vi "Handle Zoom on GPU.vi"(7 "FFT Size / 2 in":u64, 8 "error in (no error)":errorcluster, 9 "element":T1 {"Zoom Parameters"."fwidth:" format="%#_6p"; "Zoom Parameters"."f0:" format="%#_6p"}, 10 "df":dbl, 11 "Unzoomed Data In":refnum<class "2D Array f32.lvclass">) -> (0 "error out":errorcluster, 1 "Zoomed Size":u64, 2 "f0:":dbl, 3 "Zoomed Data Out":refnum<class "2D Array f32.lvclass">)   [LabVIEW 2020, in "GPU FFT Calculator.lvlib" / "GPU FFT Calculator.lvclass"]
uses:
  GPU FFT Calculator.lvclass
  GPU Calculation Message.ctl
  <vilib>/Natan Biesmans/G2CPU GPU and CPU HPC Toolkit/G2CPU Libraries/Async IO/DMA Manager/DMA Manager.lvclass
  <vilib>/Natan Biesmans/G2CPU GPU and CPU HPC Toolkit/G2CPU Libraries/Arrays/1DArray/s16/1D Array s16.lvclass
  <vilib>/Natan Biesmans/G2CPU GPU and CPU HPC Toolkit/G2CPU Libraries/Arrays/1DArray/f32/1D Array f32.lvclass
  chart zoom.ctl
  GPU Metrics.ctl
  <vilib>/Natan Biesmans/G2CPU GPU and CPU HPC Toolkit/G2CPU Libraries/Arrays/2DArray/f32/2D Array f32.lvclass
  C:/Program Files/National Instruments/LabVIEW 2026/vi.lib/Natan Biesmans/G2CPU GPU and CPU HPC Toolkit/G2CPU Libraries/Arrays/Array/Array Prototype.lvclass
  <vilib>/Natan Biesmans/G2CPU GPU and CPU HPC Toolkit/G2CPU Libraries/Arrays/Array/Array Prototype.lvclass/Array Prototype.ctl
  8252e44e-a382-477c-9ca7-689a626c88eb.vi
  e1576fc2-ceb6-43a4-8527-5ba273ea8d14.vi
  ddde6bd1-7626-4236-9c85-82b4f95f97b4.vi
  8252e44e-a382-477c-9ca7-689a626c88eb.vi/ab6cfe59-c8ad-4da3-839b-8d02ec9e015f.vi
  <vilib>/Natan Biesmans/G2CPU GPU and CPU HPC Toolkit/G2CPU Libraries/Arrays/Array/G2CPU Get Array Pointer.vi
  e1576fc2-ceb6-43a4-8527-5ba273ea8d14.vi/5793b77b-c002-4ebf-9075-685617c95341.vi
  e1576fc2-ceb6-43a4-8527-5ba273ea8d14.vi/2ed3ef86-c00d-4d71-b84c-20267a6dfcf9.vi
  ddde6bd1-7626-4236-9c85-82b4f95f97b4.vi/2e03f477-51b7-4ba0-bb4f-4f838f6557e6.vi
  ddde6bd1-7626-4236-9c85-82b4f95f97b4.vi/125d45d4-836b-469d-8a4a-6adb452f866d.vi
  ddde6bd1-7626-4236-9c85-82b4f95f97b4.vi/8038e9ed-2e71-4568-91ba-0d873494c5ed.vi
  8252e44e-a382-477c-9ca7-689a626c88eb.vi/ab6cfe59-c8ad-4da3-839b-8d02ec9e015f.vi/313ec8c5-c203-475c-9de0-0583f6fb8b4d.vi
  e1576fc2-ceb6-43a4-8527-5ba273ea8d14.vi/5793b77b-c002-4ebf-9075-685617c95341.vi/3e802c67-fb96-46a3-ae13-4994a8508b4f.vi
  e1576fc2-ceb6-43a4-8527-5ba273ea8d14.vi/5793b77b-c002-4ebf-9075-685617c95341.vi/5a50fc67-79e7-4972-80c2-92243cd53dd4.vi
  e1576fc2-ceb6-43a4-8527-5ba273ea8d14.vi/5793b77b-c002-4ebf-9075-685617c95341.vi/1c928fc9-710a-40e7-8c4f-08a1069452ae.vi
  e1576fc2-ceb6-43a4-8527-5ba273ea8d14.vi/2ed3ef86-c00d-4d71-b84c-20267a6dfcf9.vi/730f6c57-5c0b-4ee9-b61e-75067b25222b.vi
  e1576fc2-ceb6-43a4-8527-5ba273ea8d14.vi/2ed3ef86-c00d-4d71-b84c-20267a6dfcf9.vi/096b8799-7810-404e-baca-ba9279cec4bd.vi
  e1576fc2-ceb6-43a4-8527-5ba273ea8d14.vi/2ed3ef86-c00d-4d71-b84c-20267a6dfcf9.vi/0f1a5a47-bcc5-4796-ac31-8dfcfbc0d7d1.vi
  e1576fc2-ceb6-43a4-8527-5ba273ea8d14.vi/2ed3ef86-c00d-4d71-b84c-20267a6dfcf9.vi/89f12e17-3330-4b72-ad8f-8dd636660732.vi
  ddde6bd1-7626-4236-9c85-82b4f95f97b4.vi/2e03f477-51b7-4ba0-bb4f-4f838f6557e6.vi/d8e2d9cc-c923-495e-b121-b6b84788c73f.vi
  ddde6bd1-7626-4236-9c85-82b4f95f97b4.vi/2e03f477-51b7-4ba0-bb4f-4f838f6557e6.vi/345e91f0-9a5e-4de4-af9c-133346717e4a.vi
  <vilib>/Natan Biesmans/G2CPU GPU and CPU HPC Toolkit/ArrayFire Driver/VIs/Run as Multi Device.vi
  e1576fc2-ceb6-43a4-8527-5ba273ea8d14.vi/5793b77b-c002-4ebf-9075-685617c95341.vi/3e802c67-fb96-46a3-ae13-4994a8508b4f.vi/1b7cf390-2ae0-48f3-9bce-03c57eed6ee8.vi
  <vilib>/Natan Biesmans/G2CPU GPU and CPU HPC Toolkit/G2CPU Libraries/Arrays/1DArray/u32/1D Array u32.lvclass
  <vilib>/Natan Biesmans/G2CPU GPU and CPU HPC Toolkit/G2CPU Libraries/Arrays/1DArray/s32/1D Array s32.lvclass
  <vilib>/Natan Biesmans/G2CPU GPU and CPU HPC Toolkit/ArrayFire Driver/VIs/range.vi
  <vilib>/Natan Biesmans/G2CPU GPU and CPU HPC Toolkit/G2CPU Libraries/Arrays/Array/G2CPU Set Array Pointer.vi
  <vilib>/Natan Biesmans/G2CPU GPU and CPU HPC Toolkit/ArrayFire Driver/subvi/Error Converter (ErrCode or Status).vi
  <vilib>/Natan Biesmans/G2CPU GPU and CPU HPC Toolkit/G2CPU Libraries/Arrays/SubVI/is 1D.vi
  <vilib>/Natan Biesmans/G2CPU GPU and CPU HPC Toolkit/ArrayFire Driver/VIs/add.vi
  <vilib>/Natan Biesmans/G2CPU GPU and CPU HPC Toolkit/ArrayFire Driver/VIs/cast.vi
  <vilib>/Natan Biesmans/G2CPU GPU and CPU HPC Toolkit/ArrayFire Driver/VIs/lookup.vi
  <vilib>/Natan Biesmans/G2CPU GPU and CPU HPC Toolkit/G2CPU Libraries/Arrays/DataTypes/U32/U32.lvclass
  <vilib>/Natan Biesmans/G2CPU GPU and CPU HPC Toolkit/G2CPU Libraries/Arrays/1DArray/1D Array Prototype.lvclass
  <vilib>/Natan Biesmans/G2CPU GPU and CPU HPC Toolkit/G2CPU Libraries/Arrays/Array/Array Prototype.lvclass
  <vilib>/Natan Biesmans/G2CPU GPU and CPU HPC Toolkit/G2CPU Libraries/Arrays/DataTypes/I32/s32.lvclass
  Simple UI/Simple UI/Simple UI.lvclass
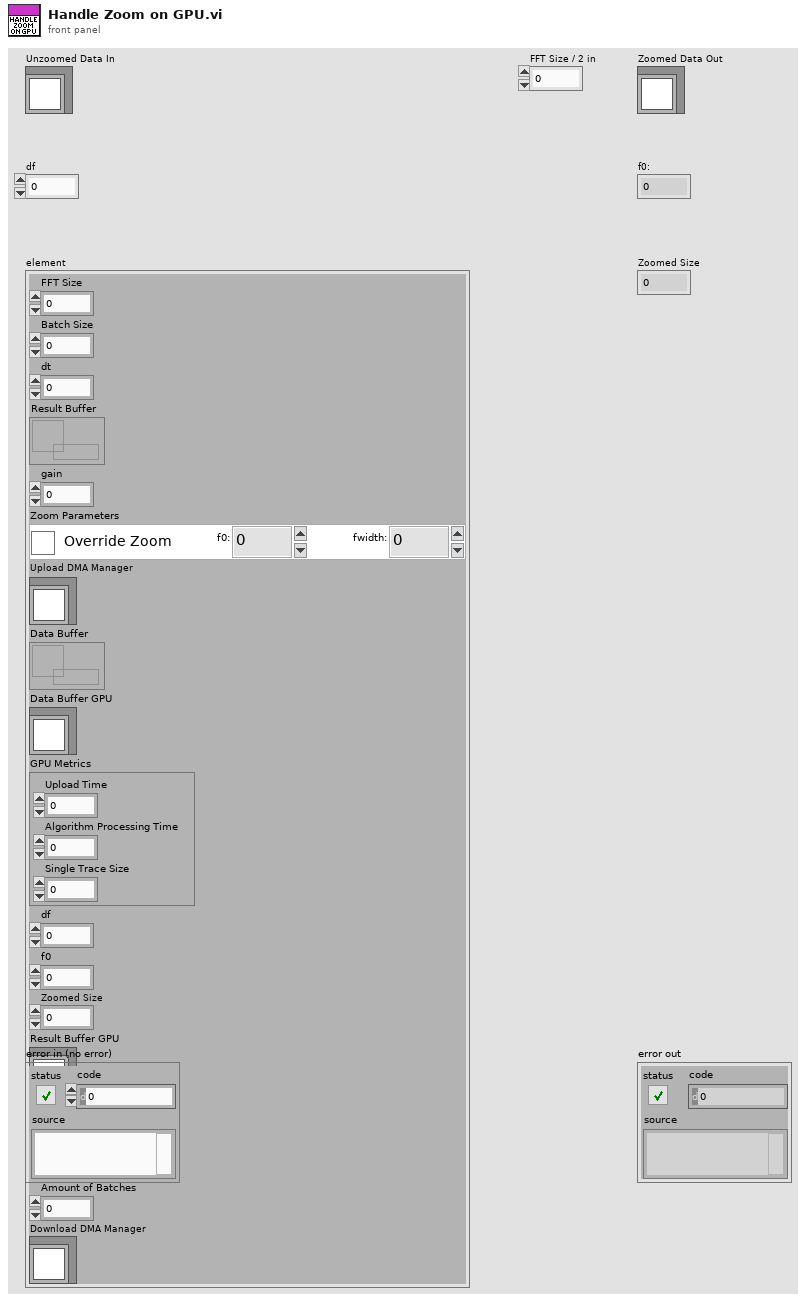
[diagram p1: front panel]
types:
  T1 = typedef "GPU FFT Calculator.lvlib/GPU FFT Calculator.lvclass/GPU Calculation Message.ctl" = cluster{"FFT Size":u64, "Batch Size":u64, "dt":dbl, "Result Buffer":refnum<data-value>, "gain":dbl, "Zoom Parameters":T2, "Upload DMA Manager":refnum<class "DMA Manager.lvclass">, "Data Buffer":refnum<data-value>, "Data Buffer GPU":refnum<class "1D Array s16.lvclass">, "GPU Metrics":T3, "df":dbl, "f0":dbl, "Zoomed Size":u64, "Result Buffer GPU":refnum<class "1D Array f32.lvclass">, "Start Time":dbl, "Batch Index":i32, "Amount of Batches":i32, "Download DMA Manager":refnum<class "DMA Manager.lvclass">}
  T2 = typedef "Simple UI.lvlib/Simple UI.lvclass/chart zoom.ctl" = cluster{"Override":bool, "f0: ":dbl, "fwidth: ":dbl}
  T3 = typedef "GPU FFT Calculator.lvlib/GPU FFT Calculator.lvclass/GPU Metrics.ctl" = cluster{"Upload Time":dbl, "Algorithm Processing Time":dbl, "Single Trace Size":u64}
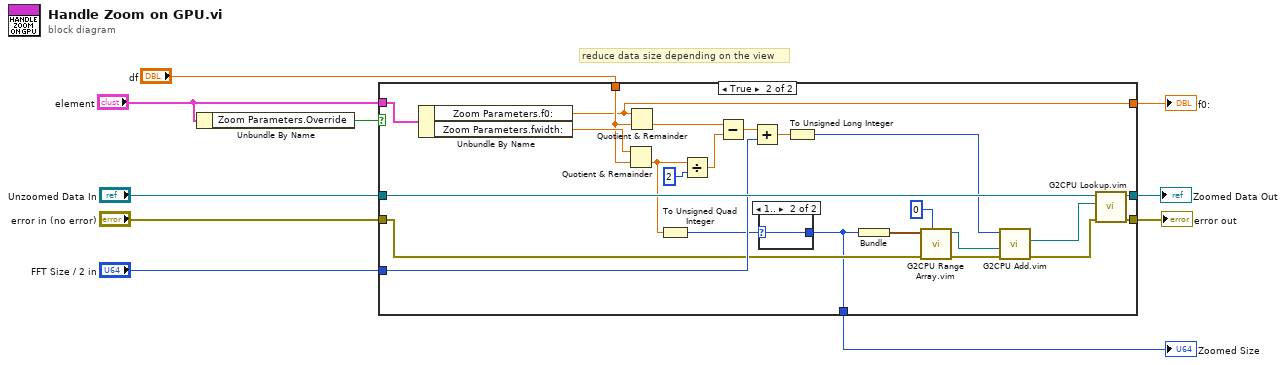
[diagram p0: block diagram]
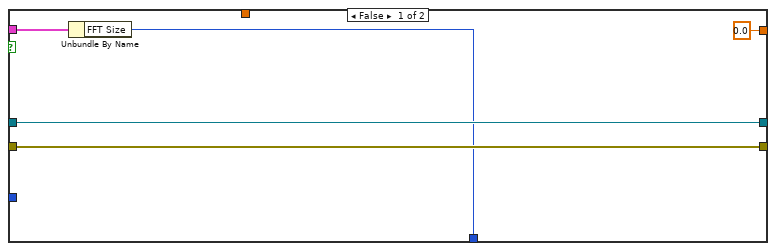
[diagram p2: hidden frame]
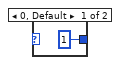
[diagram p3: hidden frame]
diagram:
  # "reduce data size depending on the view"
  n1 = Unbundle By Name("element") -> ("Zoom Parameters.Override"=w5:bool)
  n2 = case shown="True" w5 {
    tunnel: "Unzoomed Data In" -> [w15 w39]
    tunnel: "error in (no error)" -> [w14 w26]
    tunnel: [w15 w38] -> w3
    tunnel: [w14 w37] -> w4
    tunnel: "element" -> [w12 w31]
    tunnel: "df" -> [_ w30]
    tunnel: "FFT Size / 2 in" -> [_ w29]
    tunnel: [0.0 ("f0:") w18] -> w9
    tunnel: [w11 w16] -> w10
    frame False {
      n3 = Unbundle By Name(w12) -> ("FFT Size"=w11:u64)
    }
    frame True {
      n4 = Unbundle By Name(w31) -> ("Zoom Parameters.f0:"=w18:dbl, "Zoom Parameters.fwidth:"=w32:dbl)
      n5 = Quotient & Remainder(x=w32, y=w30) -> (floor(x/y)=w28:dbl)  [unwired: 1 out]
      n6 = Quotient & Remainder(x=w18, y=w30) -> (floor(x/y)=w33:dbl)  [unwired: 1 out]
      n7 = To Unsigned Quad Integer(1:w28) -> (0:w17:u64)
      n8 = Divide(x=w28, y=2) -> (x/y=w36:dbl)
      n9 = Subtract(x=w33, y=w36) -> (x-y=w35:dbl)
      n10 = Add(x=w35, y=w29) -> (x+y=w22:dbl)
      n11 = case shown="1.." w17 {
        selector: w17 -> [_ w41]
        tunnel: [u64 1 w41] -> w16
        frame 0, Default {
        }
        frame 1.. {
        }
      }
      n12 = To Unsigned Long Integer(number=w22) -> (unsigned 32bit integer=w21:u32)
      n13 = Bundle(w16) -> (w27:cluster{u64})  [unwired: 1 in]
      n14 = call "G2CPU Range Array.vim"("Datatype"=u32 0, "Error in"=w26, "Size"=w27) -> ("error out"=w25:errorcluster, "Array out"=w24:refnum<class "1D Array u32.lvclass">)  [unwired: 7 in]
      n15 = call "G2CPU Add.vim"("error in (no error)"=w25, "Array rhs"=w24, "Array lhs"=w21) -> ("error out"=w19:errorcluster, "Array Result"=w20:refnum<class "1D Array u32.lvclass">)  [unwired: 7 in]
      n16 = call "G2CPU Lookup.vim"("error in (no error)"=w19, "Indices (1D)"=w20, "Array In"=w39) -> ("error out"=w37:errorcluster, "Indexed Array"=w38:refnum<class "2D Array f32.lvclass">)  [unwired: 7 in]
    }
  }
  "Zoomed Size" <- w10
  "f0:" <- w9
  "error out" <- w4
  "Zoomed Data Out" <- w3
